vi "zmq_socket_monitor.vi"(8 "error in":errorcluster, 9 "endpoint in":string, 10 "filter (all events)":T1[](array[typedef]), 11 "socket in":refnum<class "Socket.lvclass">) -> (0 "error out":errorcluster, 1 "endpoint out":string, 2 "mask":i32, 3 "socket out":refnum<class "Socket.lvclass">)   [LabVIEW 2025, in "ZeroMQ.lvlib" / "Socket.lvclass"]
doc: "Sets up a socket monitor which checks for events on the input socket, and posts them to the provided endpoint (which should be on the inproc protocol). Only events matching the given type will be passed on.\n\nOnce the monitor has been started, a ZMQ_PAIR socket should be connected to the endpoint and will receive binary information about the events. The zmq_get_monitor_event.vi is provided to decode this information into readable form.\n\nDetailed API documentation: http://api.zeromq.org/3-2:zmq-socket-monitor"
uses:
  Socket.lvclass
  Socket.lvclass/Socket.ctl
  libzmq-v143-mt-4_3_6/LibZMQ.lvlib
  monitor_event.ctl
  ZeroMQ.lvlib
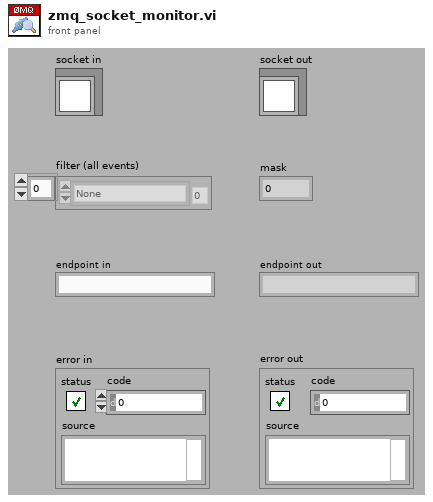
[diagram p1: front panel]
types:
  T1 = typedef "ZeroMQ.lvlib/monitor_event.ctl" = enum8{"None", "Connected", "Connect Delayed", "Connect Retry", "Listening", "Bind Failed", "Accepted", "Accept Failed", "Closed", "Close Failed", "Disconnected", "Monitor Stopped"}
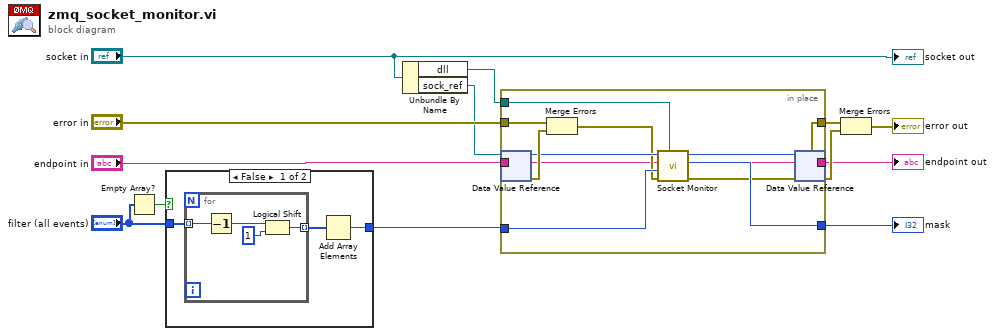
[diagram p0: block diagram]
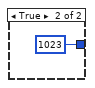
[diagram p2: hidden frame]
diagram:
  n1 = Empty Array?(array="filter (all events)") -> (empty?=w9:bool)
  n2 = case shown="False" w9 {
    tunnel: "filter (all events)" -> [w16 _]
    tunnel: [w14 1023] -> w7
    frame False {
      n3 = for {
        tunnel: w16 -> [w20] mode=indexing
        tunnel: [w17] -> w15 mode=indexing
        n4 = Decrement(x=w20) -> (x-1=w19:T1)
        n5 = Logical Shift(y=w19, x=1) -> (x << y=w17:i32)
      }
      n6 = Add Array Elements(numeric array=w15) -> (sum=w14:i32)
    }
    frame True {
    }
  }
  n7 = Unbundle By Name("socket in") -> ("dll"=w2:path, "sock_ref"=w10:refnum<data-value>)
  n8 = in-place {
    in-place-border: "endpoint in" -> [w22]
    in-place-border: "error in" -> [w31]
    in-place-border: [w23] -> w5
    in-place-border: w7 -> [w29]
    in-place-border: [w26] -> w6
    in-place-border: w2 -> [w24]
    in-place-border: [w22] -> w1
    n9 = in-place-dvr #1(w10) -> (w28:u64, w30:errorcluster)
    n10 = Merge Errors(w31, w30) -> (w25:errorcluster)
    n11 = call "Socket Monitor.vi"("path override"=w24, "error in (no error)"=w25, "events_"=w29, "addr_"=w22, "s_"=w28) -> ("error out"=w23:errorcluster, "function return"=w26:i32, "s_ out"=w27:u32)  [unwired: 4 in]
    n12 = in-place-dvr #1(w27) -> (w4:errorcluster)  [unwired: 1 out]
  }
  "endpoint out" <- w1
  "mask" <- w6
  n13 = Merge Errors(w5, w4) -> (→"error out":errorcluster)
  "socket out" <- "socket in"
